vi "ProdaNG.TestValue.New.vi"(8 "error in (no error)":errorcluster, 10 "TestValue":T1 {"minimum" format="%#.3f"; "maximum" format="%#.3f"}, 11 "dbHandleIn":i32) -> (0 "error out":errorcluster, 2 "TestValue out":T1 {"minimum" format="%#.3f"; "maximum" format="%#.3f"}, 3 "dbHandle":i32)   [LabVIEW 2016]
doc: "This function returns a product structure for a product, which is identified by a part and a serial number.\nImportant information: The field 'individual' was taken over from the field 'allgemein' of the legacy data directly. Because of this most products have the value 0 further on and only a few the value 1. \nParameter:\nhandle is an Integer, which is returned by the function Login() at the creation of a new connection.\nwabcoPartId is the Id of the part.\nserialNumber is the serial number of the product for the part above.\nproduct is a pointer on a product structure, which is filled if the returncode is 0. The structure must be defined in the calling program.\n\nReturncodes:\n0 No error\n< 0 ORACLE Error code\n6 (ERROR_INVALID_HANDLE) in case of an invalid handle\n1403 Record does not exist"
uses:
  Controls/ProdaNG.TestValue.ctl
  Controls/ProdaNG.TestValueSize.ctl
  prodllNG.dll
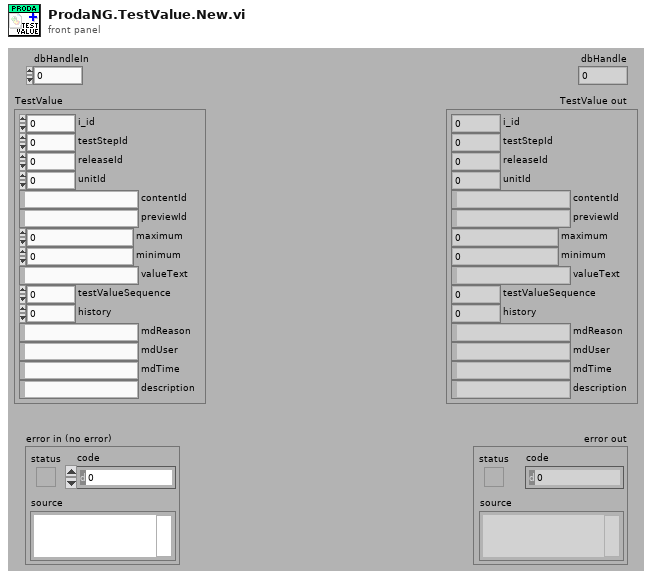
[diagram p1: front panel]
types:
  T1 = typedef "ProdaNG.TestValue.ctl" = cluster{"i_id":i32, "testStepId":i32, "releaseId":i32, "unitId":i32, "contentId":string, "previewId":string, "maximum":dbl, "minimum":dbl, "valueText":string, "testValueSequence":i32, "history":i32, "mdReason":string, "mdUser":string, "mdTime":string, "description":string}
  T2 = typedef "ProdaNG.TestValueSize.ctl" = cluster{"i_id":i32, "testStepId":i32, "releaseId":i32, "unitId":i32, "contentId":i32, "previewId":i32, "maximum":i32, "minimum":i32, "valueText":i32, "testValueSequence":i32, "history":i32, "mdReason":i32, "mdUser":i32, "mdTime":i32, "description":i32}
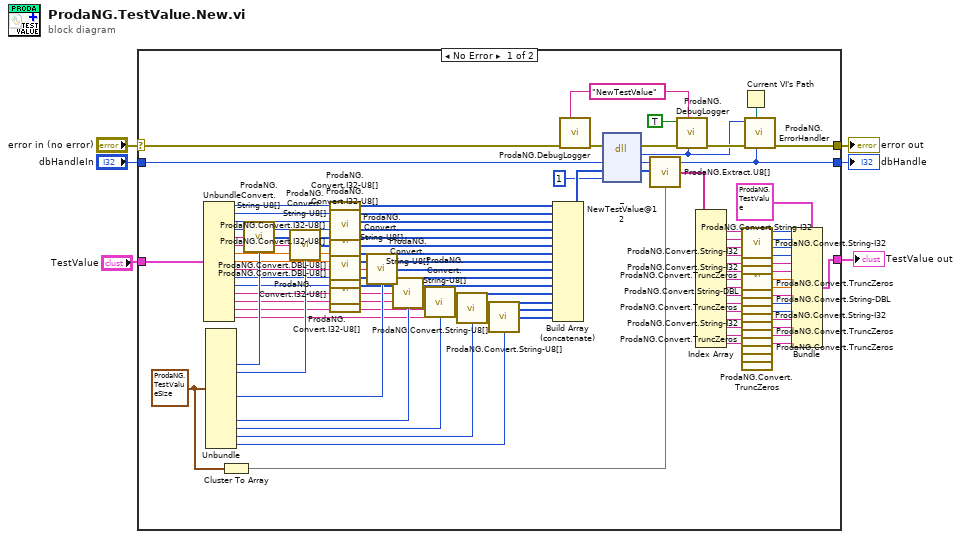
[diagram p0: block diagram]
diagram:
  n1 = case shown="No Error" "error in (no error)" {
    selector: "error in (no error)" -> [w88 w95]
    tunnel: [w93 w95] -> w5
    tunnel: "dbHandleIn" -> [w90 w94]
    tunnel: [w91 w94] -> w3
    tunnel: "TestValue" -> [w57 _]
    tunnel: [w45 _] -> w2
    frame No Error {
      w29 = T2 {"i_id"=4, "testStepId"=4, "releaseId"=4, "unitId"=4, "contentId"=16, "previewId"=16, "maximum"=8, "minimum"=8, "valueText"=258, "testValueSequence"=4, "history"=4, "mdReason"=514, "mdUser"=22, "mdTime"=24, "description"=514} ("TestStepValueSize")
      w84 = "NewTestValue" ("cmd")
      n2 = Unbundle(w57) -> ("i_id"=w80:i32, "testStepId"=w81:i32, "releaseId"=w53:i32, "unitId"=w52:i32, "contentId"=w78:string, "previewId"=w49:string, "maximum"=w28:dbl, "minimum"=w27:dbl, "valueText"=w25:string, "testValueSequence"=w22:i32, "history"=w21:i32, "mdReason"=w18:string, "mdUser"=w16:string, "mdTime"=w12:string, "description"=w11:string)
      n3 = Unbundle(w29) -> ("contentId"=w75:i32, "previewId"=w48:i32, "valueText"=w23:i32, "mdReason"=w17:i32, "mdUser"=w13:i32, "mdTime"=w9:i32, "description"=w10:i32)  [unwired: 8 out]
      n4 = Cluster To Array(cluster=w29) -> (array=w54:i32[])
      n5 = call "ProdaNG.Convert.String-U8[].vi"("Input String"=w78, "Size"=w75) -> ("Output"=w77:u8[])
      n6 = call "ProdaNG.Convert.String-U8[].vi"("Input String"=w49, "Size"=w48) -> ("Output"=w46:u8[])
      n7 = call "ProdaNG.Convert.I32-U8[].vi"("32bit integer"=w80) -> ("unsigned byte array"=w79:u8[])  [unwired: 10 in]
      n8 = call "ProdaNG.Convert.I32-U8[].vi"("32bit integer"=w81) -> ("unsigned byte array"=w82:u8[])  [unwired: 10 in]
      n9 = call "ProdaNG.Convert.I32-U8[].vi"("32bit integer"=w53) -> ("unsigned byte array"=w50:u8[])  [unwired: 10 in]
      n10 = call "ProdaNG.Convert.I32-U8[].vi"("32bit integer"=w52) -> ("unsigned byte array"=w51:u8[])  [unwired: 10 in]
      n11 = call "ProdaNG.Convert.DBL-U8[].vi"("dbl"=w28) -> ("unsigned byte array"=w76:u8[])  [unwired: 10 in]
      n12 = call "ProdaNG.Convert.DBL-U8[].vi"("dbl"=w27) -> ("unsigned byte array"=w26:u8[])  [unwired: 10 in]
      n13 = call "ProdaNG.Convert.I32-U8[].vi"("32bit integer"=w22) -> ("unsigned byte array"=w20:u8[])  [unwired: 10 in]
      n14 = call "ProdaNG.Convert.I32-U8[].vi"("32bit integer"=w21) -> ("unsigned byte array"=w19:u8[])  [unwired: 10 in]
      n15 = call "ProdaNG.Convert.String-U8[].vi"("Input String"=w25, "Size"=w23) -> ("Output"=w24:u8[])
      n16 = call "ProdaNG.Convert.String-U8[].vi"("Input String"=w18, "Size"=w17) -> ("Output"=w14:u8[])
      n17 = call "ProdaNG.Convert.String-U8[].vi"("Input String"=w16, "Size"=w13) -> ("Output"=w15:u8[])
      n18 = call "ProdaNG.Convert.String-U8[].vi"("Input String"=w12, "Size"=w9) -> ("Output"=w8:u8[])
      n19 = call "ProdaNG.Convert.String-U8[].vi"("Input String"=w11, "Size"=w10) -> ("Output"=w7:u8[])
      n20 = Build Array (concatenate)(w79, w82, w50, w51, w77, w46, w76, w26, w24, w20, w19, w14, w15, w8, w7) -> (w56:u8[])
      n21 = call "ProdaNG.DebugLogger.vi"("cmd"=w84, "error in (no error)"=w88) -> ("error out"=w87:errorcluster)  [unwired: 9 in]
      n22 = dll-call lib="D:/svn/LineTraceSystem/SOFTWARE/sources/Database/ProdaNG/prodllNG.dll" fn="_NewTestValue@12" ("ProDLL wrapper.dll:ProDLL_wrapper_GetWabcoParts_GetData")(error in=w87, "dbHandle"=w90, "testValuePtr"=w56, "doCommit"=u32 1) -> (error out=w86:errorcluster, "return type"=w83:i32, "dbHandle"=w91:i32, "testValuePtr"=w55:u8[])  [unwired: 3 in, 1 out]
      n23 = call "ProdaNG.Extract.U8[].vi"("unsigned byte array"=w55, "Sizes"=w54) -> ("Elements"=w74:string[])
      n24 = call "ProdaNG.DebugLogger.vi"("return type"=w83, "cmd"=w84, "error in (no error)"=w86, "done? (F)"=TRUE) -> ("error out"=w85:errorcluster)  [unwired: 7 in]
      n25 = Index Array(array=w74) -> (element #1=w73:string, element #2=w70:string, element #3=w69:string, element #4=w63:string, element #5=w60:string, element #6=w59:string, element #7=w64:string, element #8=w66:string, element #9=w43:string, element #10=w42:string, element #11=w41:string, element #12=w38:string, element #13=w36:string, element #14=w34:string, element #15=w33:string)  [unwired: 15 in]
      n26 = Current VI's Path() -> (path=w92:path)
      n27 = call "ProdaNG.Convert.String-I32.vi"("unsigned byte string"=w73) -> ("32bit integer"=w72:i32)  [unwired: 10 in]
      n28 = call "ProdaNG.Convert.String-I32.vi"("unsigned byte string"=w70) -> ("32bit integer"=w71:i32)  [unwired: 10 in]
      n29 = call "ProdaNG.Convert.String-I32.vi"("unsigned byte string"=w69) -> ("32bit integer"=w68:i32)  [unwired: 10 in]
      n30 = call "ProdaNG.Convert.String-I32.vi"("unsigned byte string"=w63) -> ("32bit integer"=w62:i32)  [unwired: 10 in]
      n31 = call "ProdaNG.Convert.TruncZeros.vi"("string with \\0s"=w60) -> ("LV string"=w61:string)  [unwired: 10 in]
      n32 = call "ProdaNG.Convert.TruncZeros.vi"("string with \\0s"=w59) -> ("LV string"=w58:string)  [unwired: 10 in]
      n33 = call "ProdaNG.Convert.String-DBL.vi"("unsigned byte string"=w64) -> ("dbl integer"=w65:dbl)  [unwired: 10 in]
      n34 = call "ProdaNG.Convert.String-DBL.vi"("unsigned byte string"=w66) -> ("dbl integer"=w67:dbl)  [unwired: 10 in]
      n35 = call "ProdaNG.Convert.TruncZeros.vi"("string with \\0s"=w43) -> ("LV string"=w44:string)  [unwired: 10 in]
      n36 = call "ProdaNG.Convert.String-I32.vi"("unsigned byte string"=w42) -> ("32bit integer"=w40:i32)  [unwired: 10 in]
      n37 = call "ProdaNG.Convert.String-I32.vi"("unsigned byte string"=w41) -> ("32bit integer"=w39:i32)  [unwired: 10 in]
      n38 = call "ProdaNG.Convert.TruncZeros.vi"("string with \\0s"=w38) -> ("LV string"=w37:string)  [unwired: 10 in]
      n39 = call "ProdaNG.Convert.TruncZeros.vi"("string with \\0s"=w36) -> ("LV string"=w35:string)  [unwired: 10 in]
      n40 = call "ProdaNG.Convert.TruncZeros.vi"("string with \\0s"=w34) -> ("LV string"=w32:string)  [unwired: 10 in]
      n41 = call "ProdaNG.Convert.TruncZeros.vi"("string with \\0s"=w33) -> ("LV string"=w31:string)  [unwired: 10 in]
      n42 = call "ProdaNG.ErrorHandler.vi"("dbHandleIn"=w91, "Path"=w92, "error in"=w85, "output_parameter"=w83) -> ("error out"=w93:errorcluster)  [unwired: 7 in]
      n43 = Bundle(cluster=T1 {"i_id"=0, "testStepId"=0, "releaseId"=0, "unitId"=0, "contentId"="", "previewId"="", "maximum"=0.0, "minimum"=0.0, "valueText"="", "testValueSequence"=0, "history"=0, "mdReason"="", "mdUser"="", "mdTime"="", "description"=""} ("TestStepValue"), "i_id"=w72, "testStepId"=w71, "releaseId"=w68, "unitId"=w62, "contentId"=w61, "previewId"=w58, "maximum"=w65, "minimum"=w67, "valueText"=w44, "testValueSequence"=w40, "history"=w39, "mdReason"=w37, "mdUser"=w35, "mdTime"=w32, "description"=w31) -> (w45:T1)
    }
    frame Error {
    }
  }
  "error out" <- w5
  "dbHandle" <- w3
  "TestValue out" <- w2
